vi "WebServices Base URL--constant.vi"() -> (3 "WebServices Base URL":string)   [LabVIEW 2020, in "WSsupport.lvlib"]
uses:
  WSsupport.lvlib
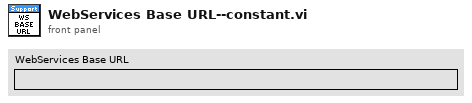
[diagram p1: front panel]
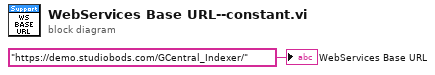
[diagram p0: block diagram]
diagram:
  "WebServices Base URL" <- "https://demo.studiobods.com/GCentral_Indexer/"
